vi "PC_Main.vi"() -> ()   [LabVIEW 2018]
uses:
  <vilib>/rvi/Analysis/host/Butterworth/config/Butterworth Filter Order.ctl
  <vilib>/rvi/Analysis/host/Butterworth/config/Butterworth Filter Type.ctl
  <vilib>/Analysis/1siggen.llb/Ramp Pattern by Samples.vi
  <vilib>/Analysis/2dsp.llb/Power Spectrum (DBL).vi
  <vilib>/Utility/file.llb/Write Delimited Spreadsheet (string).vi
  <vilib>/Utility/file.llb/Write Delimited Spreadsheet (DBL).vi
  <vilib>/rvi/Analysis/host/Butterworth/config/BwScaledCoefficients.vi
  <vilib>/rvi/errors/niLvFpgaErrorClusterFromErrorCode.vi
  <vilib>/rvi/Analysis/host/Notch/config/NotchScaledCoefficients.vi
  <vilib>/rvi/Analysis/host/Butterworth/XNode/ButterworthCoefficients.xnode
  <vilib>/rvi/Analysis/host/Notch/XNode/NotchCoefficients.xnode
  <vilib>/Analysis/NI_AALBase.lvlib
  <vilib>/Analysis/NI_AALPro.lvlib
  <vilib>/rvi/Analysis/host/Public/NI_FpgaMspHost.lvlib
panel:
  in  "delay (us)":dbl=8.4
  in  "B3 f (kHz)":dbl=20.0 caption="f (kHz)"
  in  "B1 f (kHz)":dbl=4.0 caption="f (kHz)"
  in  "N bw (kHz)":dbl=14.0 caption="bw (kHz)"
  in  "N f (kHz)":dbl=12.0 caption="f (kHz)"
  in  "B2 f (kHz)":dbl=4.0 caption="f (kHz)"
  in  "f2 (kHz)":dbl=32.0
  in  "f1 (kHz)":dbl=20.0
  in  "auto reset":bool
  out "ADC\nOverflow":bool
  out "Gain \ntoo high":bool
  in  "target ampl.":dbl=6.0 min=0.0 max=9.5
  in  "set auto gain":bool
  in  "Gain":fxp<+,20,8>=1.0
  in  "Pause Button":bool
  in  "refresh rate (Hz)":dbl=10.0
  out "std phase 2":dbl caption="std(ph) (deg)" format="%0.2f"
  out "mean phase 2":dbl caption="phase (deg)" format="%0.2f"
  out "mean freq 2":dbl caption="f (Hz)" format="%0.2f"
  out "std freq 2":dbl caption="std(f) (Hz)" format="%0.2f"
  in  "min std(f) (Hz)":dbl=10.0
  in  "filename":string="test"
  in  "Save":bool caption="Blank Button"
  out "saved as":path
  in  "Plot everything":bool=TRUE
  in  "store ratio":i16=4
  in  "base freq 2 (Hz)":fxp<+,18,17>=32000.0
  in  "Tab Control":T1(tab)=enum."Frequency"
  out "Spectrum":T2(graph)
  out "ADC in":cluster{dbl[], dbl[]}(graph)
  in  "scope idx":u8=1 min=1 max=3
  out "Phase PLL1":cluster{dbl[], dbl[]}(graph)
  out "Phase PLL2":cluster{dbl[], dbl[]}(graph)
  out "Delta Frequency PLL1":cluster{dbl[], dbl[]}(graph)
  out "Delta Frequency PLL2":cluster{dbl[], dbl[]}(graph)
  out "Frequency Spectrum PLL1":cluster{dbl[], dbl[]}(graph)
  out "Frequency Spectrum PLL2":cluster{dbl[], dbl[]}(graph)
  in  "reset":bool
  in  "I gain":fxp<+,20,6>=6.5
  in  "P gain":fxp<+,14,14>=2000.0
  in  "base freq 1 (Hz)":fxp<+,18,17>=20000.0
  out "std phase 1":dbl caption="std(ph) (deg)" format="%0.2f"
  out "mean phase 1":dbl caption="phase (deg)" format="%0.2f"
  out "mean freq 1":dbl caption="f (Hz)" format="%0.2f"
  out "std freq 1":dbl caption="std(f) (Hz)" format="%0.2f"
  in  "Stop":bool
  in  "Stop RT":bool
  # "FPGA PLL - PC Main"
  # "Gain Settings"
  # "PLL Settings"
  # "Warnings"
  # "PLL 1"
  # "PLL 2"
  # "Filter Settings"
  # "Low-Pass"
  # "Band-Stop"
  # "1"
  # "2"
  # "3"
  # "Live Scope"
  # "Save Data"
  # "t (ms)"
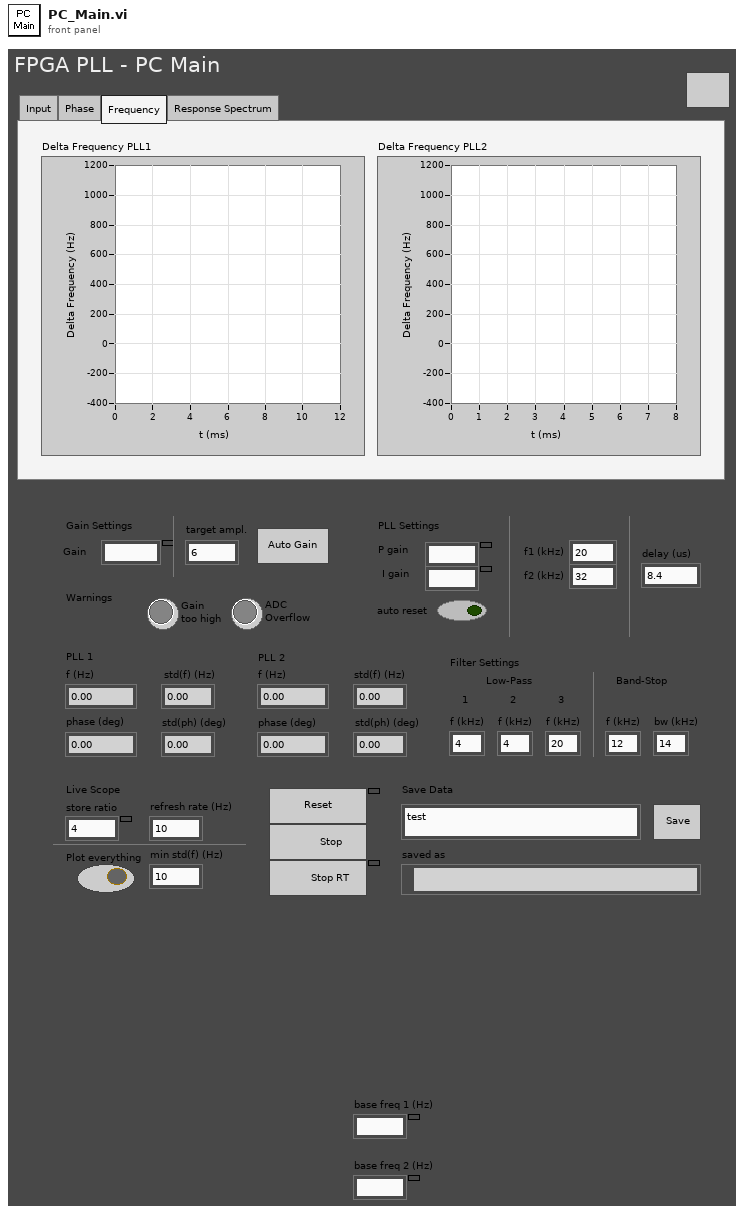
[diagram p1: front panel]
types:
  T1 = enum32{"Input", "Phase", "Frequency", "Response Spectrum"}
  T2 = cluster{"Ramp Pattern":dbl[], "Power Spectrum":dbl[]}[]
  T3 = cluster{"scaled coefficients":i32[], "channel index":u16}
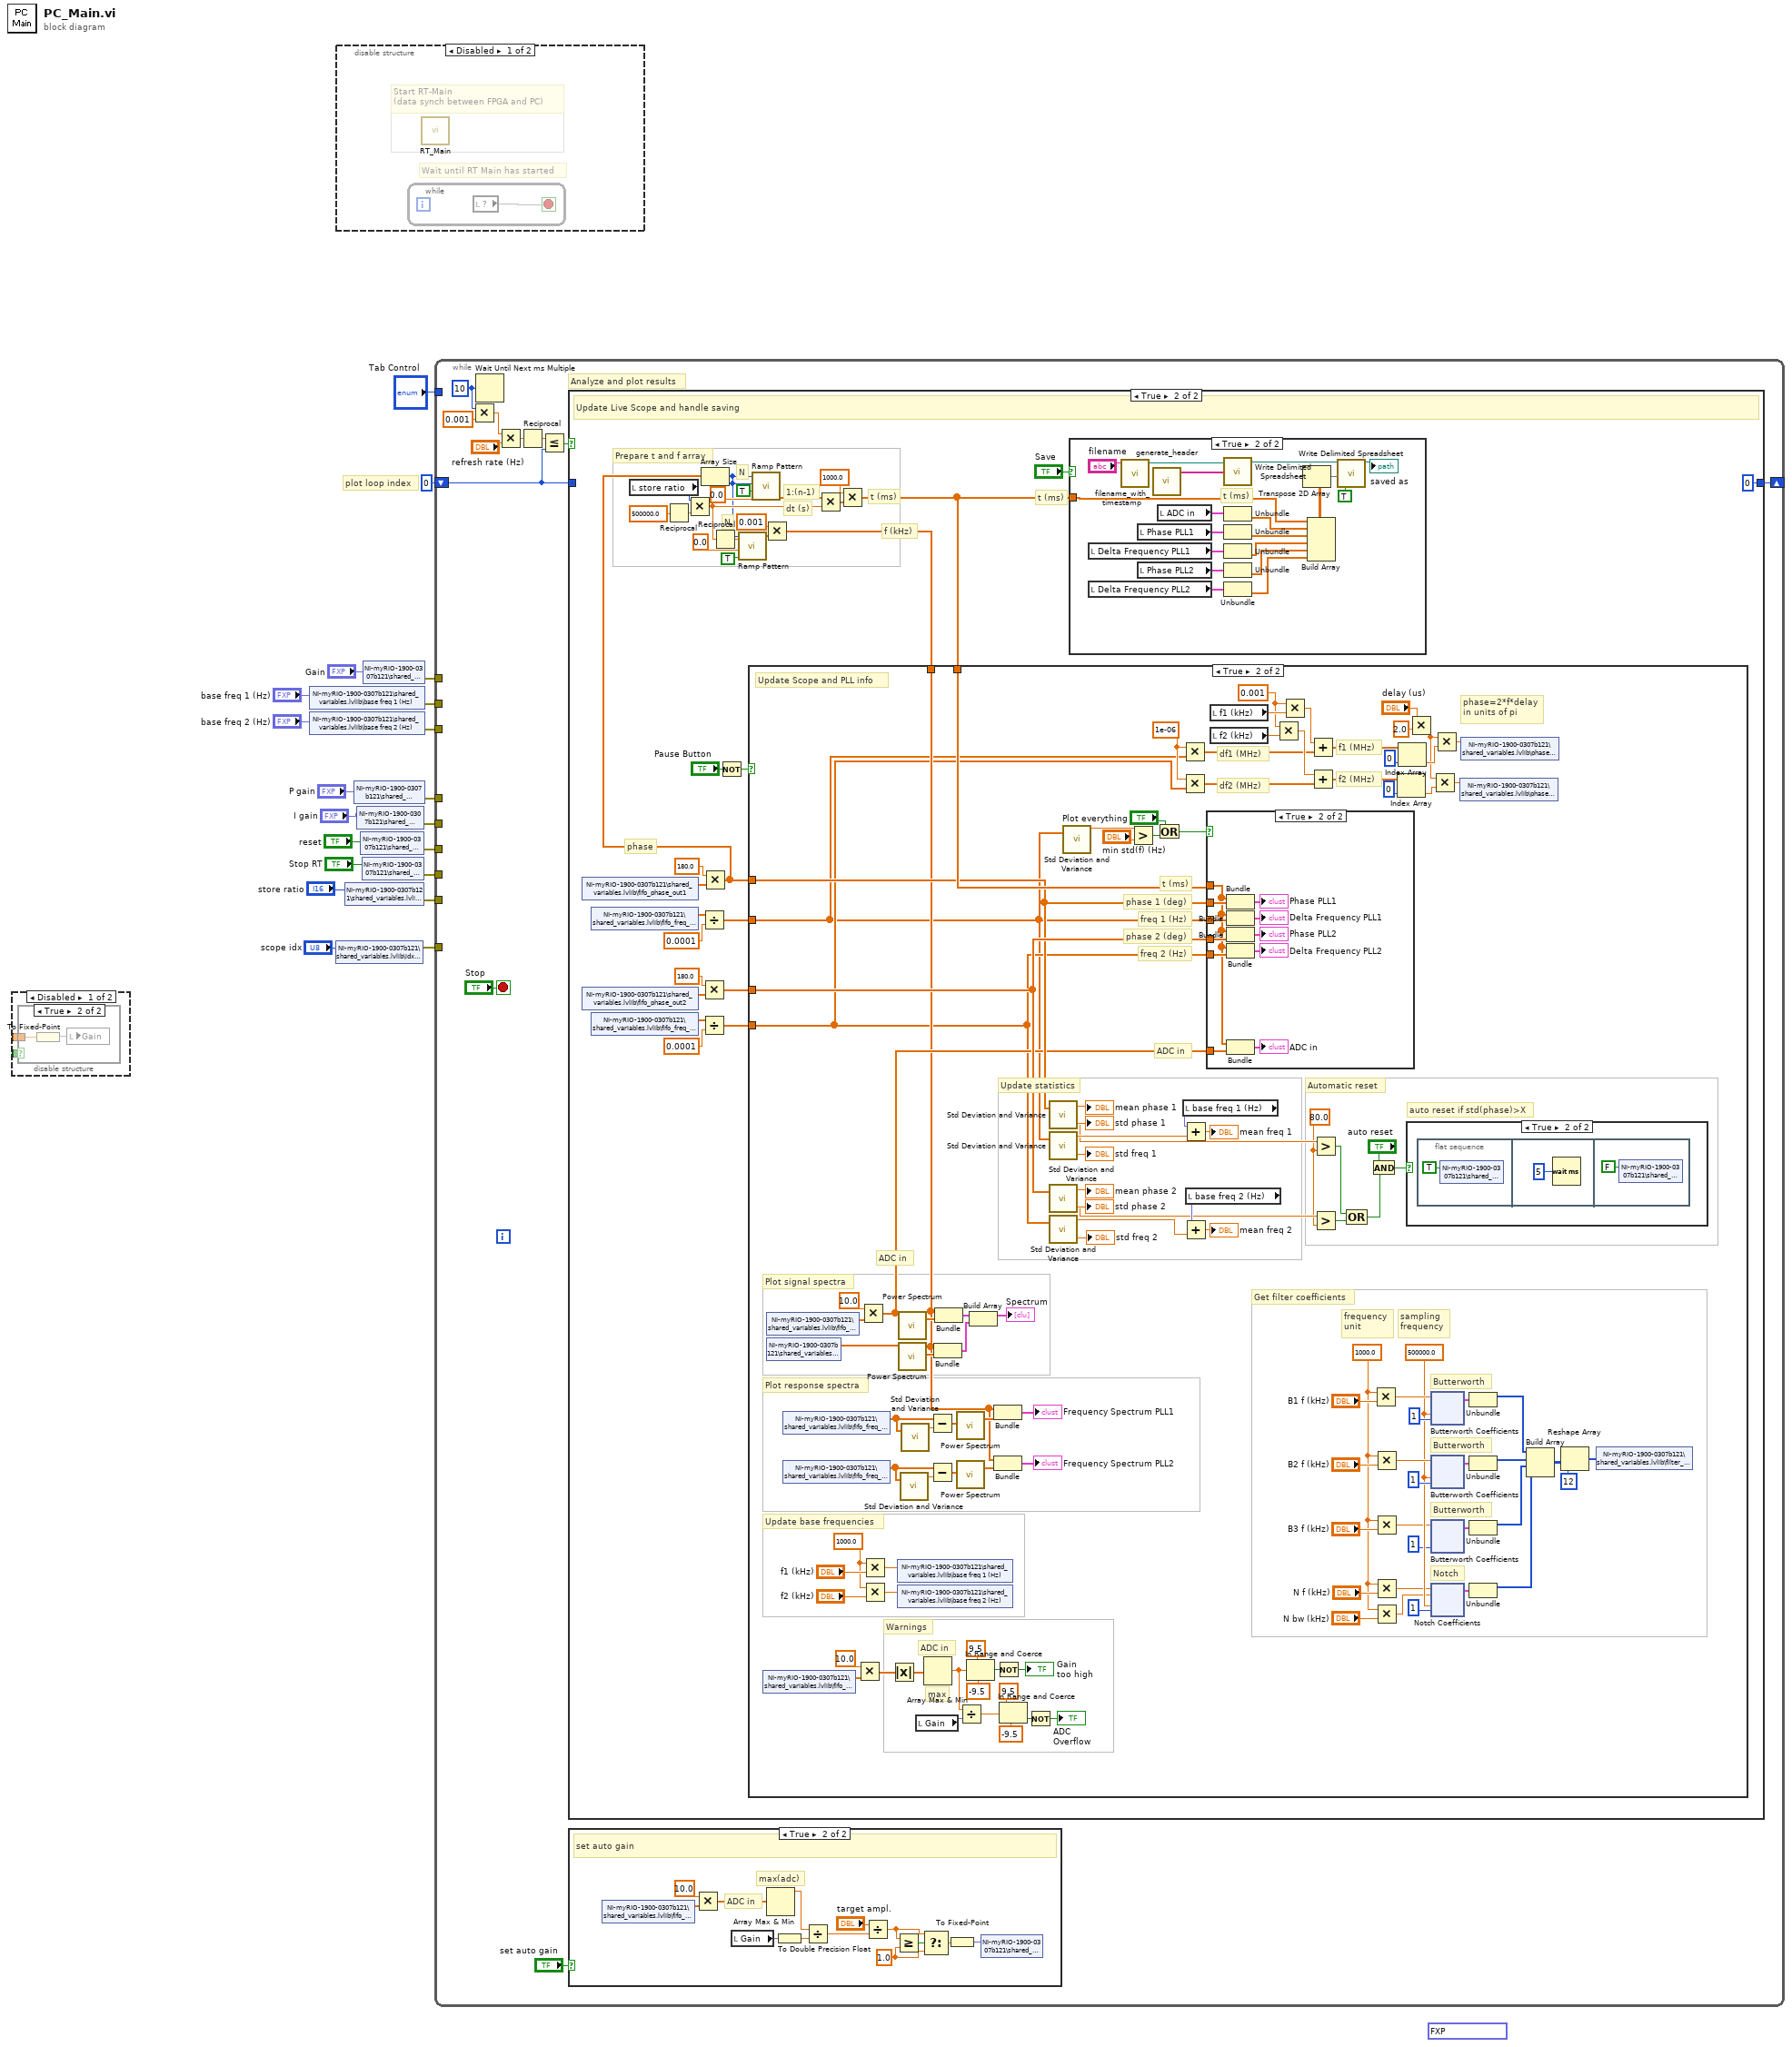
[diagram p0: block diagram]
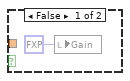
[diagram p2: hidden frame]
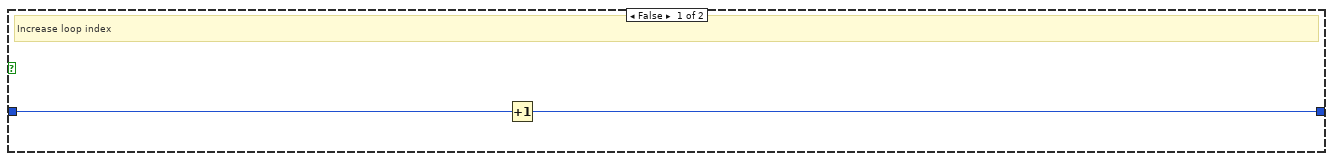
[diagram p5: hidden frame]
diagram:
  (unwired) fxp<+,12,0> 0.000244140625 ("y")
  # "plot loop index"
  n1 = disable-structure shown="Disabled" {
    disable-tunnel: _ -> [w22 _]
    disable-tunnel: _ -> [w21 _]
    frame Disabled {
      n2 = case shown="True" w21 {
        tunnel: w22 -> [_ w24]
        frame False {
          n3 = local write "Gain"(fxp<+,20,8> 1.0 ("Gain")) -> ()
        }
        frame True {
          n4 = To Fixed-Point(number=w24) -> (fixed-point=w25:fxp<+,20,8>)  [unwired: 1 in]
          n5 = local write "Gain"(w25) -> ()
        }
      }
    }
    frame Enabled {
    }
  }
  n6 = shared-variable "NI-myRIO-1900-0307b121\\shared_variables.lvlib\\base freq 1 (Hz)"("base freq 1 (Hz)") -> (error out=w18:errorcluster)  [unwired: 1 in]
  n7 = shared-variable "NI-myRIO-1900-0307b121\\shared_variables.lvlib\\base freq 2 (Hz)"("base freq 2 (Hz)") -> (error out=w3:errorcluster)  [unwired: 1 in]
  n8 = shared-variable "NI-myRIO-1900-0307b121\\shared_variables.lvlib\\idx_scope"("scope idx") -> (error out=w1:errorcluster)  [unwired: 1 in]
  n9 = disable-structure shown="Disabled" {
    frame Disabled {
      # "Wait until RT Main has started"
      # "Start RT-Main \n(data synch between FPGA and PC)"
      n10 = while {
        stop <- w26 stop-if-true
        n11 = local read item#-1() -> (w26)
      }
      n12 = call "RT_Main.vi"() -> ()  [unwired: 11 in, 1 out]
    }
    frame Enabled {
    }
  }
  n13 = shared-variable "NI-myRIO-1900-0307b121\\shared_variables.lvlib\\idx_pick"("store ratio") -> (error out=w10:errorcluster)  [unwired: 1 in]
  n14 = shared-variable "NI-myRIO-1900-0307b121\\shared_variables.lvlib\\P gain"("P gain") -> (error out=w17:errorcluster)  [unwired: 1 in]
  n15 = shared-variable "NI-myRIO-1900-0307b121\\shared_variables.lvlib\\I gain"("I gain") -> (error out=w16:errorcluster)  [unwired: 1 in]
  n16 = shared-variable "NI-myRIO-1900-0307b121\\shared_variables.lvlib\\reset"("reset") -> (error out=w14:errorcluster)  [unwired: 1 in]
  n17 = shared-variable "NI-myRIO-1900-0307b121\\shared_variables.lvlib\\stop"("Stop RT") -> (error out=w12:errorcluster)  [unwired: 1 in]
  n18 = shared-variable "NI-myRIO-1900-0307b121\\shared_variables.lvlib\\gain"("Gain") -> (error out=w5:errorcluster)  [unwired: 1 in]
  n19 = while {
    tunnel: w18 -> [_]
    tunnel: w17 -> [_]
    tunnel: w16 -> [_]
    tunnel: w14 -> [_]
    tunnel: w12 -> [_]
    tunnel: w10 -> [_]
    tunnel: "Tab Control" -> [_]
    shift-right: [w29] -> _
    shift-left: u32 0 -> [w28]
    tunnel: w5 -> [_]
    tunnel: w3 -> [_]
    tunnel: w1 -> [_]
    stop <- "Stop" stop-if-true
    w33 = u32 10 ("millisecond multiple")
    # "Analyze and plot results"
    n20 = Multiply(x=w33, y=0.001 ("x")) -> (x*y=w32:dbl)
    n21 = Wait Until Next ms Multiple(millisecond multiple=w33) -> ()  [unwired: 1 out]
    n22 = Multiply(x=w32, y="refresh rate (Hz)") -> (x*y=w30:dbl)
    n23 = Reciprocal(x=w30) -> (1/x=w31:dbl)
    n24 = Less Or Equal?(x=w31, y=w28) -> (x <= y?=w37:bool)
    n25 = case shown="True" w37 {
      tunnel: w28 -> [w51 _]
      tunnel: [w52 u32 0] -> w29
      frame False {
        # "Increase loop index"
        n26 = Increment(x=w51) -> (x+1=w52:u32)
      }
      frame True {
        # "t (ms)"
        # "f (kHz)"
        # "t (ms)"
        # "phase"
        # "Prepare t and f array"
        # "N"
        # "N"
        # "dt (s)"
        # "1:(n-1)"
        # "Update Live Scope and handle saving"
        n27 = shared-variable "NI-myRIO-1900-0307b121\\shared_variables.lvlib\\fifo_phase_out1"() -> (w84:dbl[])  [unwired: 1 in, 1 out]
        n28 = shared-variable "NI-myRIO-1900-0307b121\\shared_variables.lvlib\\fifo_phase_out2"() -> (w70:dbl[])  [unwired: 1 in, 1 out]
        n29 = shared-variable "NI-myRIO-1900-0307b121\\shared_variables.lvlib\\fifo_freq_out1"() -> (w81:dbl[])  [unwired: 1 in, 1 out]
        n30 = shared-variable "NI-myRIO-1900-0307b121\\shared_variables.lvlib\\fifo_freq_out2"() -> (w53:dbl[])  [unwired: 1 in, 1 out]
        n31 = local read "store ratio"() -> (w79:i16)
        n32 = Reciprocal(x=500000.0) -> (1/x=w78:dbl)
        n33 = Multiply(x=w79, y=w78) -> (x*y=w62:dbl)
        n34 = Divide(x=w81, y=0.0001 ("x")) -> (x/y=w67:dbl[])
        n35 = Multiply(x=180.0, y=w70) -> (x*y=w68:dbl[])
        n36 = Divide(x=w53, y=0.0001 ("x")) -> (x/y=w66:dbl[])
        n37 = Multiply(x=180.0, y=w84) -> (x*y=w54:dbl[])
        n38 = Array Size(array=w54) -> (size(s)=w60:i32)
        n39 = Reciprocal(x=w62) -> (1/x=w61:dbl)
        n40 = Not(x="Pause Button") -> (.not. x?=w55:bool)
        n41 = call-poly <vilib>:"Ramp Pattern.vi"("exclude end?"=TRUE, "start"=0.0, "end"=w61, "samples"=w60) -> ("Ramp Pattern"=w59:dbl[])  [unwired: 6 in, 1 out]
        n42 = call-poly <vilib>:"Ramp Pattern.vi"("exclude end?"=TRUE, "start"=0.0, "end"=w60, "samples"=w60) -> ("Ramp Pattern"=w69:dbl[])  [unwired: 6 in, 1 out]
        n43 = Multiply(x=0.001 ("start"), y=w59) -> (x*y=w57:dbl[])
        n44 = Multiply(x=w69, y=w62) -> (x*y=w73:dbl[])
        n45 = Multiply(x=1000.0, y=w73) -> (x*y=w65:dbl[])
        n46 = case shown="True" w55 {
          tunnel: w68 -> [_ w190]
          tunnel: w67 -> [_ w86]
          tunnel: w66 -> [_ w87]
          tunnel: w65 -> [_ w189]
          tunnel: w54 -> [_ w188]
          tunnel: w57 -> [_ w134]
          frame False {
          }
          frame True {
            w95 = 1e-06
            w98 = 0.001
            w109 = 1000.0 ("sample rate (S/s)")
            w123 = 500000.0 ("sample rate (S/s)")
            w143 = 1000.0 ("x")
            w142 = 80.0 ("y")
            # "df2 (MHz)"
            # "df1 (MHz)"
            # "phase=2*f*delay\nin units of pi"
            # "f1 (MHz)"
            # "f2 (MHz)"
            # "Butterworth"
            # "Notch"
            # "Get filter coefficients"
            # "Butterworth"
            # "Butterworth"
            # "frequency\nunit"
            # "sampling\nfrequency"
            # "Automatic reset"
            # "Update statistics"
            # "Update base frequencies"
            # "auto reset if std(phase)>X"
            # "Plot response spectra"
            # "Warnings"
            # "ADC in"
            # "max"
            # "Update Scope and PLL info"
            # "ADC in"
            # "Plot signal spectra"
            # "ADC in"
            # "freq 2 (Hz)"
            # "phase 2 (deg)"
            # "t (ms)"
            # "freq 1 (Hz)"
            # "phase 1 (deg)"
            n47 = shared-variable "NI-myRIO-1900-0307b121\\shared_variables.lvlib\\fifo_adc_in"() -> (w166:dbl[])  [unwired: 1 in, 1 out]
            n48 = shared-variable "NI-myRIO-1900-0307b121\\shared_variables.lvlib\\fifo_adc_in"() -> (w167:dbl[])  [unwired: 1 in, 1 out]
            n49 = shared-variable "NI-myRIO-1900-0307b121\\shared_variables.lvlib\\fifo_ref"() -> (w137:dbl[])  [unwired: 1 in, 1 out]
            n50 = shared-variable "NI-myRIO-1900-0307b121\\shared_variables.lvlib\\fifo_freq_out1"() -> (w159:dbl[])  [unwired: 1 in, 1 out]
            n51 = shared-variable "NI-myRIO-1900-0307b121\\shared_variables.lvlib\\fifo_freq_out2"() -> (w156:dbl[])  [unwired: 1 in, 1 out]
            n52 = Multiply(x=10.0, y=w166) -> (x*y=w150:dbl[])
            n53 = Multiply(x=10.0, y=w167) -> (x*y=w177:dbl[])
            n54 = Multiply(x=w143, y="f1 (kHz)") -> (x*y=w147:dbl)
            n55 = Multiply(x=w143, y="f2 (kHz)") -> (x*y=w144:dbl)
            n56 = Absolute Value(x=w150) -> (abs(x)=w149:dbl[])
            n57 = shared-variable "NI-myRIO-1900-0307b121\\shared_variables.lvlib\\base freq 1 (Hz)"(w147) -> ()  [unwired: 1 in, 1 out]
            n58 = shared-variable "NI-myRIO-1900-0307b121\\shared_variables.lvlib\\base freq 2 (Hz)"(w144) -> ()  [unwired: 1 in, 1 out]
            n59 = call-poly <vilib>:"Power Spectrum.vi"("X"=w177) -> ("Power Spectrum"=w191:dbl[])  [unwired: 1 out]
            n60 = call-poly <vilib>:"Power Spectrum.vi"("X"=w137) -> ("Power Spectrum"=w136:dbl[])  [unwired: 1 out]
            n61 = call <vilib>:"Std Deviation and Variance.vi"("X"=w156) -> ("mean"=w157:dbl)  [unwired: 1 in, 2 out]
            n62 = call <vilib>:"Std Deviation and Variance.vi"("X"=w159) -> ("mean"=w160:dbl)  [unwired: 1 in, 2 out]
            n63 = local read "Gain"() -> (w173:fxp<+,20,8>)
            n64 = Array Max & Min(array=w149) -> (max value=w174:dbl)  [unwired: 3 out]
            n65 = Subtract(x=w159, y=w160) -> (x-y=w158:dbl[])
            n66 = Subtract(x=w156, y=w157) -> (x-y=w155:dbl[])
            n67 = Bundle(w134, "Power Spectrum"=w136) -> (w135:cluster{dbl[], "Power Spectrum":dbl[]})  [unwired: 1 in]
            n68 = Bundle(w134, "Power Spectrum"=w191) -> (w152:cluster{dbl[], "Power Spectrum":dbl[]})  [unwired: 1 in]
            n69 = call-poly <vilib>:"Power Spectrum.vi"("X"=w158) -> ("Power Spectrum"=w162:dbl[])  [unwired: 1 out]
            n70 = call-poly <vilib>:"Power Spectrum.vi"("X"=w155) -> ("Power Spectrum"=w161:dbl[])  [unwired: 1 out]
            n71 = Divide(x=w174, y=w173) -> (x/y=w171:dbl)
            n72 = In Range and Coerce(upper limit=9.5, x=w174, lower limit=-9.5) -> (In Range?=w176:bool)  [unwired: 1 out]
            n73 = Build Array(w152, w135) -> (→"Spectrum":cluster{dbl[], "Power Spectrum":dbl[]}[])
            n74 = Bundle(w134, "Power Spectrum"=w162) -> (→"Frequency Spectrum PLL1":cluster{dbl[], "Power Spectrum":dbl[]})  [unwired: 1 in]
            n75 = Bundle(w134, "Power Spectrum"=w161) -> (→"Frequency Spectrum PLL2":cluster{dbl[], "Power Spectrum":dbl[]})  [unwired: 1 in]
            n76 = Not(x=w176) -> (.not. x?=→"Gain \ntoo high":bool)
            n77 = In Range and Coerce(upper limit=9.5, x=w171, lower limit=-9.5) -> (In Range?=w168:bool)  [unwired: 1 out]
            n78 = Not(x=w168) -> (.not. x?=→"ADC\nOverflow":bool)
            n79 = call <vilib>:"Std Deviation and Variance.vi"("X"=w188) -> ("mean"=→"mean phase 1":dbl, "standard deviation"=→"std phase 1":dbl, "variance"=w153:dbl)  [unwired: 1 in]
            n80 = call <vilib>:"Std Deviation and Variance.vi"("X"=w86) -> ("mean"=w185:dbl, "standard deviation"=→"std freq 1":dbl)  [unwired: 1 in, 1 out]
            n81 = call <vilib>:"Std Deviation and Variance.vi"("X"=w190) -> ("mean"=→"mean phase 2":dbl, "standard deviation"=→"std phase 2":dbl, "variance"=w154:dbl)  [unwired: 1 in]
            n82 = call <vilib>:"Std Deviation and Variance.vi"("X"=w87) -> ("mean"=w182:dbl, "standard deviation"=→"std freq 2":dbl)  [unwired: 1 in, 1 out]
            n83 = call <vilib>:"Std Deviation and Variance.vi"("X"=w86) -> ("standard deviation"=w198:dbl)  [unwired: 1 in, 2 out]
            n84 = Greater?(x=w198, y="min std(f) (Hz)") -> (0:w196:bool)
            n85 = Or(x="Plot everything", y=w196) -> (x .or. y?=w181:bool)
            n86 = Multiply(x=w95, y=w86) -> (x*y=w94:dbl[])
            n87 = Multiply(x=w95, y=w87) -> (x*y=w93:dbl[])
            n88 = local read "base freq 1 (Hz)"() -> (w186:fxp<+,18,17>)
            n89 = Add(x=w186, y=w185) -> (x+y=→"mean freq 1":dbl)
            n90 = local read "base freq 2 (Hz)"() -> (w184:fxp<+,18,17>)
            n91 = Add(x=w184, y=w182) -> (x+y=→"mean freq 2":dbl)
            n92 = case shown="True" w181 {
              tunnel: w188 -> [_ w320]
              tunnel: w86 -> [_ w319]
              tunnel: w189 -> [_ w312]
              tunnel: w190 -> [_ w316]
              tunnel: w87 -> [_ w315]
              tunnel: w177 -> [_ w313]
              frame False {
              }
              frame True {
                n93 = Bundle(w312, w320) -> (→"Phase PLL1":cluster{dbl[], dbl[]})  [unwired: 1 in]
                n94 = Bundle(w312, w319) -> (→"Delta Frequency PLL1":cluster{dbl[], dbl[]})  [unwired: 1 in]
                n95 = Bundle(w312, w316) -> (→"Phase PLL2":cluster{dbl[], dbl[]})  [unwired: 1 in]
                n96 = Bundle(w312, w315) -> (→"Delta Frequency PLL2":cluster{dbl[], dbl[]})  [unwired: 1 in]
                n97 = Bundle(w312, w313) -> (→"ADC in":cluster{dbl[], dbl[]})  [unwired: 1 in]
              }
            }
            n98 = local read "f1 (kHz)"() -> (w100:dbl)
            n99 = local read "f2 (kHz)"() -> (w99:dbl)
            n100 = Multiply(x=w98, y=w99) -> (x*y=w97:dbl)
            n101 = Multiply(x=w98, y=w100) -> (x*y=w96:dbl)
            n102 = Add(x=w96, y=w94) -> (x+y=w92:dbl[])
            n103 = Add(x=w97, y=w93) -> (x+y=w91:dbl[])
            n104 = Greater?(x=w153, y=w142) -> (0:w140:bool)
            n105 = Greater?(x=w154, y=w142) -> (0:w139:bool)
            n106 = Compound Arithmetic op=OR(w140, w139) -> (w138:bool)
            n107 = And(x="auto reset", y=w138) -> (x .and. y?=w148:bool)
            n108 = Multiply(x=w109, y="B1 f (kHz)") -> (x*y=w131:dbl)
            n109 = Multiply(x=w109, y="B2 f (kHz)") -> (x*y=w132:dbl)
            n110 = Multiply(x=w109, y="B3 f (kHz)") -> (x*y=w110:dbl)
            n111 = Multiply(x=w109, y="N f (kHz)") -> (x*y=w121:dbl)
            n112 = Multiply(x=w109, y="N bw (kHz)") -> (x*y=w116:dbl)
            n113 = Index Array(array=w91, index=0) -> (element=w102:dbl)
            n114 = Index Array(array=w92, index=0) -> (element=w105:dbl)
            n115 = case shown="True" w148 {
              frame False {
              }
              frame True {
                n116 = flat-sequence {
                  frame #0 {
                    n117 = shared-variable "NI-myRIO-1900-0307b121\\shared_variables.lvlib\\reset"(TRUE ("reset")) -> ()  [unwired: 1 in, 1 out]
                  }
                  frame #1 {
                    n118 = Wait (ms)(milliseconds to wait=u32 5) -> ()  [unwired: 1 out]
                  }
                  frame #2 {
                    n119 = shared-variable "NI-myRIO-1900-0307b121\\shared_variables.lvlib\\reset"(FALSE ("reset")) -> ()  [unwired: 1 in, 1 out]
                  }
                }
              }
            }
            n120 = Multiply(x="delay (us)", y=2.0) -> (x*y=w101:dbl)
            n121 = Multiply(x=w101, y=w102) -> (x*y=w89:dbl)
            n122 = xnode "Butterworth Coefficients"("cutoff frequency (Hz)"=w131, "sample rate (S/s)"=w123, "channel index"=u16 1) -> ("configuration"=w128:T3)  [unwired: 1 in, 1 out]
            n123 = xnode "Butterworth Coefficients"("cutoff frequency (Hz)"=w132, "sample rate (S/s)"=w123, "channel index"=u16 1) -> ("configuration"=w129:T3)  [unwired: 1 in, 1 out]
            n124 = xnode "Butterworth Coefficients"("cutoff frequency (Hz)"=w110, "channel index"=u16 1) -> ("configuration"=w111:T3)  [unwired: 2 in, 1 out]
            n125 = xnode "Notch Coefficients"("notch frequency (Hz)"=w121, "notch width (Hz)"=w116, "sample rate (S/s)"=w123, "channel index"=u16 1) -> ("configuration"=w119:T3)  [unwired: 1 in, 1 out]
            n126 = Multiply(x=w101, y=w105) -> (x*y=w88:dbl)
            n127 = shared-variable "NI-myRIO-1900-0307b121\\shared_variables.lvlib\\phase_corr2"(w89) -> ()  [unwired: 1 in, 1 out]
            n128 = shared-variable "NI-myRIO-1900-0307b121\\shared_variables.lvlib\\phase_corr1"(w88) -> ()  [unwired: 1 in, 1 out]
            n129 = Unbundle(w128) -> ("scaled coefficients"=w124:i32[])  [unwired: 1 out]
            n130 = Unbundle(w129) -> ("scaled coefficients"=w125:i32[])  [unwired: 1 out]
            n131 = Unbundle(w111) -> ("scaled coefficients"=w108:i32[])  [unwired: 1 out]
            n132 = Unbundle(w119) -> ("scaled coefficients"=w107:i32[])  [unwired: 1 out]
            n133 = Build Array(w124, w125, w108, w107) -> (w133:i32[][])
            n134 = Reshape Array(w133, 12 ("dimension size")) -> (w120:i32[])
            n135 = shared-variable "NI-myRIO-1900-0307b121\\shared_variables.lvlib\\filter_coeffs"(w120) -> ()  [unwired: 1 in, 1 out]
          }
        }
        n136 = case shown="True" "Save" {
          tunnel: w65 -> [_ w327]
          frame False {
          }
          frame True {
            # "t (ms)"
            n137 = local read "Delta Frequency PLL1"() -> (w331:cluster{dbl[], dbl[]})
            n138 = local read "Delta Frequency PLL2"() -> (w330:cluster{dbl[], dbl[]})
            n139 = call "filename_with_timestamp.vi"("filename"="filename") -> ("filepath"=w323:path)  [unwired: 10 in]
            n140 = local read "Phase PLL1"() -> (w333:cluster{dbl[], dbl[]})
            n141 = local read "Phase PLL2"() -> (w332:cluster{dbl[], dbl[]})
            n142 = call "generate_header.vi"() -> ("header\narray"=w324:string[])  [unwired: 11 in]
            n143 = local read "ADC in"() -> (w336:cluster{dbl[], dbl[]})
            n144 = call-poly <vilib>:"Write Delimited Spreadsheet.vi"("file path (dialog if empty)"=w323, "1D data"=w324) -> ("new file path (Not A Path if cancelled)"=w325:path)  [unwired: 12 in, 1 out]
            n145 = Unbundle(w336) -> (w335:dbl[])  [unwired: 1 out]
            n146 = Unbundle(w333) -> (w334:dbl[])  [unwired: 1 out]
            n147 = Unbundle(w331) -> (w329:dbl[])  [unwired: 1 out]
            n148 = Unbundle(w332) -> (w328:dbl[])  [unwired: 1 out]
            n149 = Unbundle(w330) -> (w326:dbl[])  [unwired: 1 out]
            n150 = Build Array(w327, w335, w334, w329, w328, w326) -> (w340:dbl[][])
            n151 = Transpose 2D Array(2D array=w340) -> (transposed array=w339:dbl[][])
            n152 = call-poly <vilib>:"Write Delimited Spreadsheet.vi"("file path (dialog if empty)"=w325, "2D data"=w339, "append to file? (new file:F)"=TRUE) -> ("new file path (Not A Path if cancelled)"=→"saved as":path)  [unwired: 11 in, 1 out]
          }
        }
      }
    }
    n153 = case shown="True" "set auto gain" {
      frame False {
      }
      frame True {
        w43 = 1.0 ("y")
        # "ADC in"
        # "max(adc)"
        # "set auto gain"
        n154 = shared-variable "NI-myRIO-1900-0307b121\\shared_variables.lvlib\\fifo_adc_in"() -> (w39:dbl[])  [unwired: 1 in, 1 out]
        n155 = Multiply(x=10.0, y=w39) -> (x*y=w46:dbl[])
        n156 = local read "Gain"() -> (w50:fxp<+,20,8>)
        n157 = Array Max & Min(array=w46) -> (max value=w49:dbl)  [unwired: 3 out]
        n158 = To Double Precision Float(number=w50) -> (double precision float=w48:dbl)
        n159 = Divide(x=w49, y=w48) -> (x/y=w42:dbl)
        n160 = Divide(x="target ampl.", y=w42) -> (x/y=w40:dbl)
        n161 = Greater Or Equal?(x=w40, y=w43) -> (x >= y?=w45:bool)
        n162 = Select(t=w40, s=w45, f=w43) -> (s? t:f=w44:dbl)
        n163 = To Fixed-Point(number=w44) -> (fixed-point=w38:fxp<+,20,8>)  [unwired: 1 in]
        n164 = shared-variable "NI-myRIO-1900-0307b121\\shared_variables.lvlib\\gain"(w38) -> ()  [unwired: 1 in, 1 out]
      }
    }
  }
